vi "Demo Simple Sound.vi"(8 "error in (no error)":errorcluster) -> (0 "error out":errorcluster)   [LabVIEW 2011]
uses:
  VIremote.llb/VIremoteEvent.ctl
  VIremote.llb/VIremoteFunction.ctl
panel:
  in  "Play sample.wav":bool
  in  "Repeat":bool
  in  "stop":bool
  out "sound":i16[](graph)
  in  "Play":bool
  in  "VIremoteEvent":T1=enum."Connection Closed"
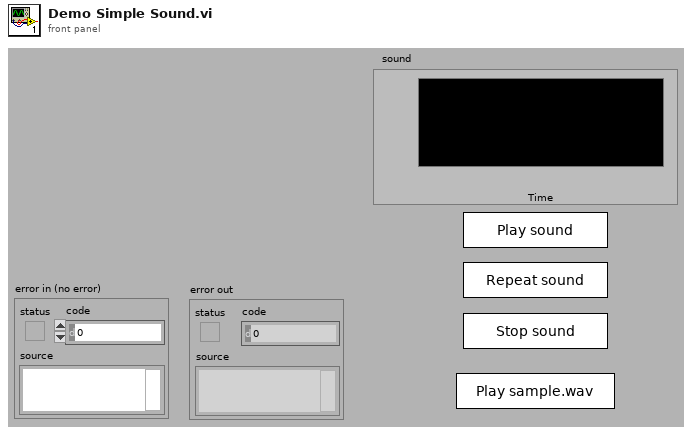
[diagram p1: front panel]
types:
  T1 = typedef "VIremoteEvent.ctl" = enum16{"No Event", "Connection Closed", "Navigate Back", "Enter Background", "Enter Foreground", "Portrait", "Portrait Upside Down", "Landscape Left", "Landscape Right"}
  T2 = enum16{"big-endian, network order", "native, host order", "little-endian"}
  T3 = typedef "VIremoteFunction.ctl" = enum16{"Do nothing", "Stop controller", "Close this connection", "Show info panel", "Set VI to control", "Set Accelerometer freq (Hz)", "Show Alert message", "Start Sound Input", "Stop Sound Input", "Set Volume (0-100)", "Set sound output Speaker", "Set sound output Receiver", "Play Sound", "Repeat Sound", "Stop Sound", "Pause Sound", "Resume Sound", "Set panel width of caller (320 or 480)", "Set Panel Size to Portrait", "Set Panel Size to Landscape", "Set Panel Size as Current Orientation", "Allow all UI Orientations", "Send user notification", "Disable Scrolling", "Normal Scrolling", "Page Scrolling", "Set Scroll Offset", "Page Indicator Position"}
  T4 = enum32{"invalid app kind", "Development System", "Run Time System", "Student Edition", "Embedded LabVIEW", "Evaluation", "Custom"}
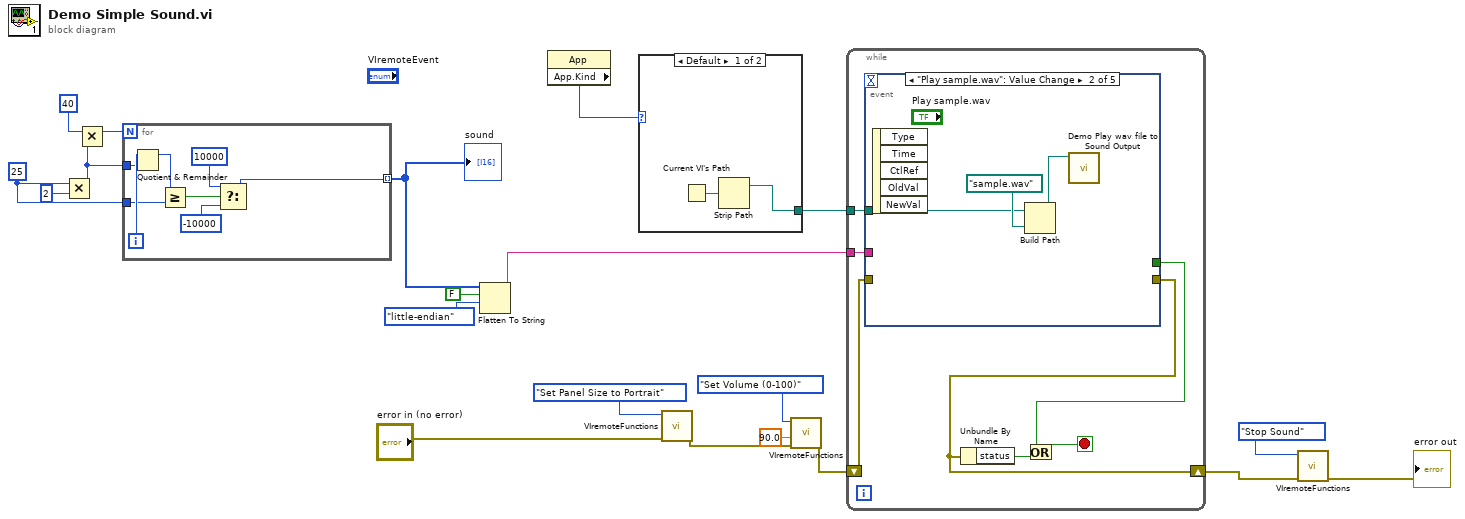
[diagram p0: block diagram]
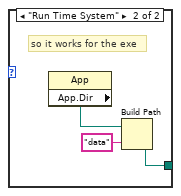
[diagram p2: hidden frame]
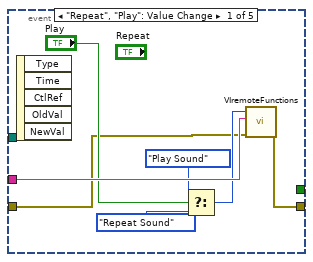
[diagram p3: hidden frame]
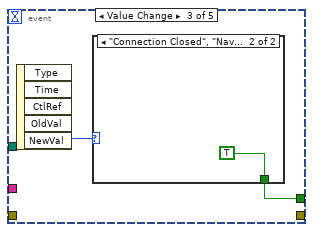
[diagram p4: hidden frame]
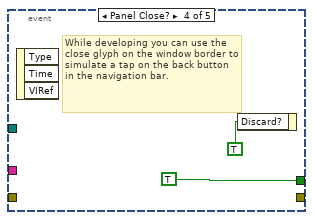
[diagram p6: hidden frame]
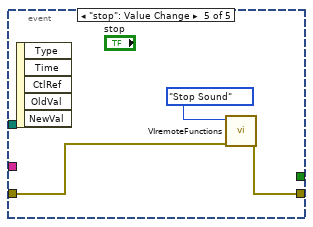
[diagram p7: hidden frame]
diagram:
  w8 = 25 ("y")
  n1 = Multiply(x=w8, y=2) -> (x*y=w9:i32)
  n2 = Multiply(x=40, y=w9) -> (x*y=w11:i32)
  n3 = for {
    N: w11 -> [_]
    tunnel: [w21] -> w5 mode=indexing
    tunnel: w9 -> [w27]
    tunnel: w8 -> [w25]
    i -> [w28]
    n4 = Quotient & Remainder(x=w28, y=w27) -> (x-y*floor(x/y)=w26:i32)  [unwired: 1 out]
    n5 = Greater Or Equal?(x=w26, y=w25) -> (x >= y?=w24:bool)
    n6 = Select(t=i16 10000 ("y"), s=w24, f=i16 -10000 ("y")) -> (s? t:f=w21:i16)
  }
  "sound" <- w5
  n7 = Flatten To String(anything=w5, prepend array or string size? (T)=FALSE, byte order (0:big-endian, network order)=T2."little-endian") -> (data string=w7:string)  [unwired: 1 in, 2 out]
  n8 = property class="App"() -> ("App.Kind"=w2:T4)  [unwired: 2 in, 2 out]
  n9 = case shown="Default" w2 {
    tunnel: [w29 w31] -> w1
    frame Default {
      n10 = Current VI's Path() -> (path=w30:path)
      n11 = Strip Path(path=w30) -> (stripped path=w29:path)  [unwired: 1 out]
    }
    frame "Run Time System" {
      # "so it works for the exe"
      n12 = property class="App"() -> ("App.Dir"=w33:path)  [unwired: 2 in, 2 out]
      n13 = Build Path(base path=w33, name or relative path="data") -> (appended path=w31:path)
    }
  }
  n14 = call "VIremoteFunctions.vi"("error in (no error)"="error in (no error)", "Function"=VIremoteFunction."Set Panel Size to Portrait") -> ("error out"=w15:errorcluster)  [unwired: 4 in, 5 out]
  n15 = call "VIremoteFunctions.vi"("error in (no error)"=w15, "Value in"=90.0, "Function"=VIremoteFunction."Set Volume (0-100)") -> ("error out"=w14:errorcluster)  [unwired: 3 in, 5 out]
  n16 = while {
    shift-right: [w38] -> w18
    shift-left: w14 -> [w37]
    tunnel: w7 -> [w36]
    tunnel: w1 -> [w34]
    stop <- w40 stop-if-true
    n17 = event shown="[1] \"Play sample.wav\": Value Change" {
      selector: _ -> [_ _ _ _ _]
      dyn-events: _ -> [_ _ _ _ _]
      timeout: _ -> [_ _ _ _ _]
      tunnel: [w42 _ _ _ w56] -> w38
      tunnel: w37 -> [w41 _ _ _ w57]
      tunnel: w36 -> [w47 _ _ _ _]
      tunnel: [_ _ w51 TRUE ("Discard?") _] -> w35
      tunnel: w34 -> [_ w48 _ _ _]
      event "Repeat", "Play": Value Change {
        n18 = event-data() -> ()  [unwired: 6 out]
        n19 = Select(t=VIremoteFunction."Play Sound" ("Function"), s="Play", f=VIremoteFunction."Repeat Sound" ("Function")) -> (s? t:f=w43:T3)
        n20 = call "VIremoteFunctions.vi"("error in (no error)"=w41, "String in"=w47, "Function"=w43) -> ("error out"=w42:errorcluster)  [unwired: 3 in, 5 out]
      }
      event "Play sample.wav": Value Change {
        n21 = event-data() -> ()  [unwired: 6 out]
        n22 = Build Path(base path=w48, name or relative path=path "sample.wav" ("File Path")) -> (appended path=w49:path)
        n23 = call "Demo Play wav file to Sound Output.vi"("File Path"=w49) -> ()  [unwired: 1 in, 10 out]
      }
      event Value Change {
        n24 = event-data() -> ("NewVal"=w52:T1)  [unwired: 5 out]
        n25 = case shown="\"Connection Closed\", \"Navigate Back\"" w52 {
          tunnel: [_ TRUE] -> w51
          frame "No Event", Default {
          }
          frame "Connection Closed", "Navigate Back" {
          }
        }
      }
      event Panel Close? {
        # "While developing you can use the close glyph on the window border to simulate a tap on the back button in the navigation bar."
        n26 = event-data() -> ()  [unwired: 4 out]
        n27 = event-data("Discard?"=TRUE) -> ()  [unwired: 1 in, 1 out]
      }
      event "stop": Value Change {
        n28 = event-data() -> ()  [unwired: 6 out]
        n29 = call "VIremoteFunctions.vi"("error in (no error)"=w57, "Function"=VIremoteFunction."Stop Sound") -> ("error out"=w56:errorcluster)  [unwired: 4 in, 5 out]
      }
    }
    n30 = Unbundle By Name(w38) -> ("status"=w39:bool)
    n31 = Or(x=w35, y=w39) -> (x .or. y?=w40:bool)
  }
  n32 = call "VIremoteFunctions.vi"("error in (no error)"=w18, "Function"=VIremoteFunction."Stop Sound") -> ("error out"=→"error out":errorcluster)  [unwired: 4 in, 5 out]
